vi "List Registered Feeds.vi"(8 "error in":errorcluster) -> (0 "error out":errorcluster, 2 "registered feeds":T1[](array[typedef]))   [LabVIEW 2014, in "NIPM_API.lvlib"]
uses:
  NIPM_API.lvlib
  _support/feed.ctl
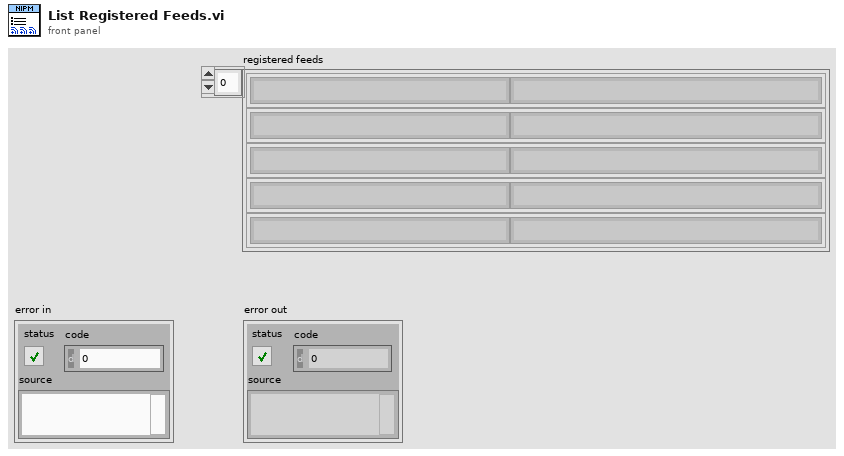
[diagram p1: front panel]
types:
  T1 = typedef "NIPM_API.lvlib/feed.ctl" = cluster{"Name":string, "URI":string}
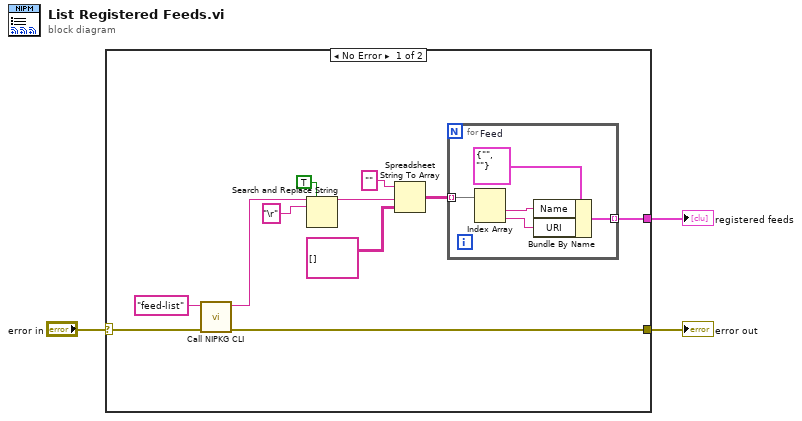
[diagram p0: block diagram]
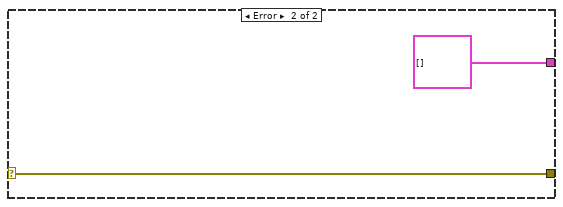
[diagram p2: hidden frame]
diagram:
  n1 = case shown="No Error" "error in" {
    selector: "error in" -> [w14 w21]
    tunnel: [w12 w21] -> w2
    tunnel: [w4 T1[] []] -> w1
    frame No Error {
      n2 = call "Call NIPKG CLI.vi"("error in (no error)"=w14, "command"="feed-list" ("format string")) -> ("error out"=w12:errorcluster, "command line standard output"=w6:string)  [unwired: 8 in]
      n3 = Search and Replace String(replace all?=TRUE ("replace all? (F)"), input string=w6, search string="\r") -> (result string=w9:string)  [unwired: 5 in, 3 out]
      n4 = Spreadsheet String To Array(format string="", spreadsheet string=w9, array type (2D Dbl)=string[][] []) -> (array=w5:string[][])  [unwired: 1 in]
      n5 = for {
        tunnel: w5 -> [w19] mode=indexing
        tunnel: [w15] -> w4 mode=indexing
        w18 = T1 {"Name"="", "URI"=""}  # Feed
        n6 = Index Array(array=w19) -> (element #1=w17:string, element #2=w16:string)  [unwired: 2 in]
        n7 = Bundle By Name(cluster=w18, "Name"=w17, "URI"=w16) -> (w15:T1)
      }
    }
    frame Error {
    }
  }
  "error out" <- w2
  "registered feeds" <- w1
